vi "cno_call objective function with scaling.vi"(5 "cno data":T1, 6 "function":enum16{"initialize", "execute"}(ring)=enum."execute", 7 "user defined functions":T2, 8 "error in (no error)":errorcluster, 9 "scale":dbl[](array[numeric]), 11 "X":dbl[](array[numeric])) -> (0 "error out":errorcluster, 1 "num function calls":i32, 3 "out":dbl[](array[numeric]))   [LabVIEW 2018, in "NI_Gmath.lvlib"]
doc: "OB=cost(P(NIC+1:NPIC).*SCALE(NC+2:NC+NP+1),0)./SCALE(1:NC+1)"
uses:
  NI_Gmath.lvlib
  cno_user defined functions.ctl
  cno_user objective function ref.ctl
  objective function data.ctl
  cno_data.ctl
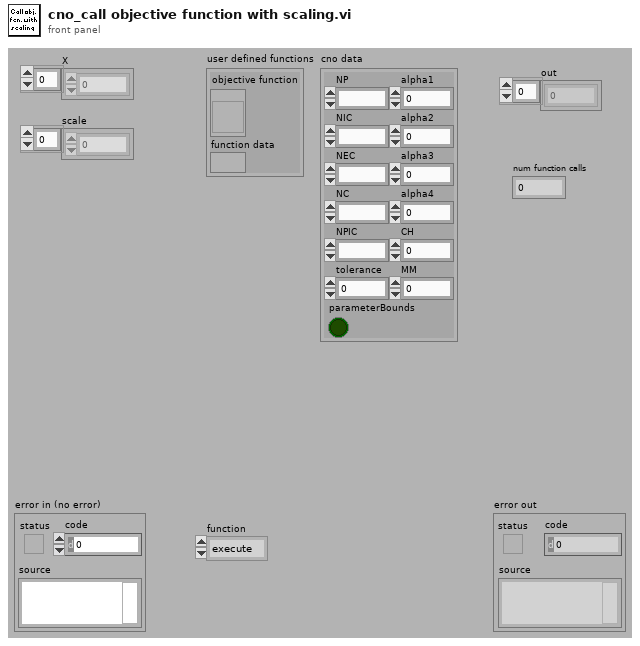
[diagram p1: front panel]
types:
  T1 = typedef "NI_Gmath.lvlib/cno_data.ctl" = cluster{"NP":i32, "NIC":i32, "NEC":i32, "NC":i32, "NPIC":i32, "parameterBounds":bool, "alpha1":dbl, "alpha2":dbl, "alpha3":dbl, "alpha4":dbl, "CH":i32, "MM":i32, "tolerance":dbl}
  T2 = typedef "NI_Gmath.lvlib/cno_user defined functions.ctl" = cluster{"objective function":T3, "function data":T4}
  T3 = typedef "NI_Gmath.lvlib/cno_user objective function ref.ctl" = refnum<vi>
  T4 = typedef "NI_Gmath.lvlib/objective function data.ctl" = variant
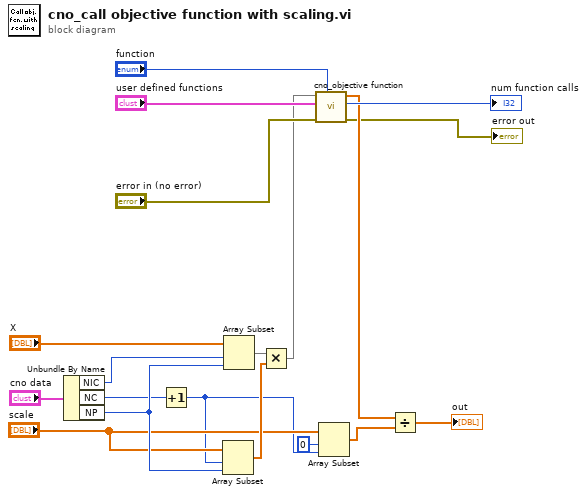
[diagram p0: block diagram]
diagram:
  n1 = Unbundle By Name("cno data") -> ("NIC"=w15:i32, "NC"=w13:i32, "NP"=w14:i32)
  n2 = Increment(x=w13) -> (x+1=w10:i32)
  n3 = Array Subset(array="scale", index=w10, length=w14) -> (w17:dbl[])
  n4 = Array Subset(array="X", index=w15, length=w14) -> (w18:dbl[])
  n5 = Multiply(x=w18, y=w17) -> (x*y=w4:dbl[])
  n6 = call "cno_objective function.vi"("function"="function", "error in (no error)"="error in (no error)", "user defined functions"="user defined functions", "X"=w4) -> ("error out"=→"error out":errorcluster, "num function calls"=→"num function calls":i32, "F(X)"=w3:dbl[])  [unwired: 5 in]
  n7 = Array Subset(array="scale", index=0, length=w10) -> (w9:dbl[])
  n8 = Divide(x=w3, y=w9) -> (x/y=→"out":dbl[])
